vi "test Custom Regex.vi"(8 "error in":errorcluster) -> (0 "error out":errorcluster)   [LabVIEW 2020, in "serenial.io-ase.test.lvlib"]
uses:
  serenial.io-ase.test.lvlib
  Custom Regex/Custom Regex.lvclass
  C:/serenial/libraries/asynchronous-system-exec/LabVIEW/serenial.io-ase/configuration/configuration.lvclass
  serenial.io-ase/ase/ase.lvclass/ase.ctl
  serenial.io-ase/ase/Start Call (Exe-Args).vi
  serenial.io-ase/ase/Start Call (Internal).vi
  serenial.io-ase/ase/Write Data to Std In.vi
  serenial.io-ase/ase/Merge Call Library Errors.vi
  serenial.io-ase/ase/NI-Linux-RT-64 Library Path.vi
  serenial.io-ase/ase/Error Empty Executable Name.vi
  serenial.io-ase/ase/Check Shared Library Version.vi
  serenial.io-ase/ase/Trim Whitespace.vi
  serenial.io-ase/ase/Error Invalid ASE Handle.vi
  serenial.io-ase/ase/Error Internal Library Implementation Error.vi
  <vilib>/Utility/error.llb/Error Cluster From Error Code.vi
  <vilib>/addons/_JKI Toolkits/Caraya/classes/Assert/Assert Equal Value and Type_Variant.vi
  serenial.io-ase/ase/ase.lvclass
  <vilib>/ErrorRing/Error Ring.xnode
  serenial.io-ase/configuration/configuration.lvclass
  <vilib>/addons/_JKI Toolkits/Caraya/classes/Test/Test.lvclass
  <vilib>/addons/_JKI Toolkits/Caraya/classes/Assert/Assert.lvclass
  C:/serenial/libraries/asynchronous-system-exec/LabVIEW/serenial.io-ase.test/Custom Regex/Custom Regex.lvclass
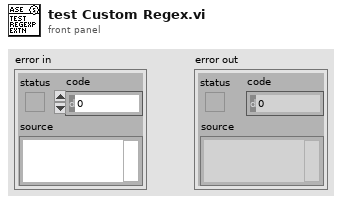
[diagram p1: front panel]
types:
  T1 = typedef "serenial.io-ase.lvlib/ase.lvclass/Event References.ctl" = cluster{"Standard Output":refnum<user-event>, "Standard Error":refnum<user-event>, "Did Exit":refnum<user-event>}
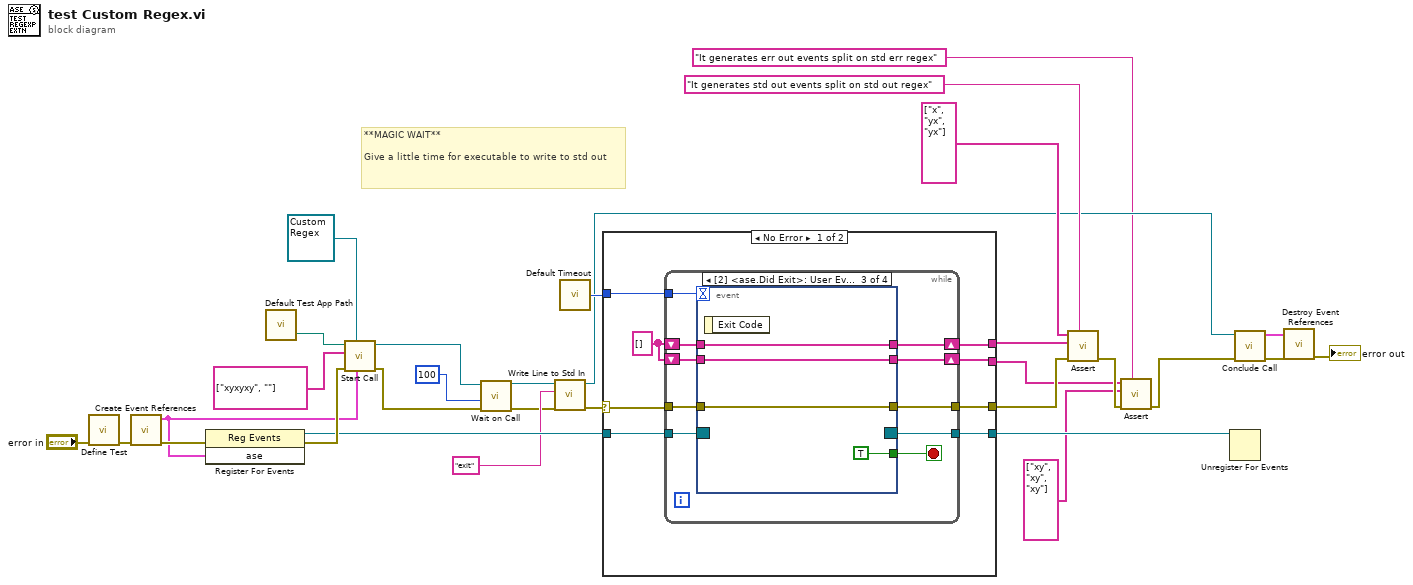
[diagram p0: block diagram]
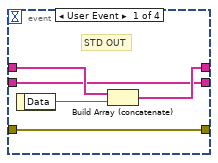
[diagram p2: hidden frame]
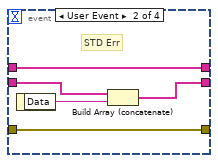
[diagram p3: hidden frame]
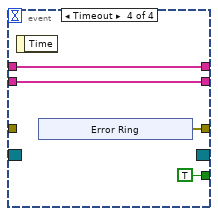
[diagram p4: hidden frame]
diagram:
  # "**MAGIC WAIT**\n\nGive a little time for executable to write to std out"
  n1 = call <vilib>:"Define Test.vi"("error in (no error)"="error in") -> ("error out"=w29:errorcluster)  [unwired: 10 in]
  n2 = call "Create Event References.vi"("error in"=w29) -> ("error out"=w31:errorcluster, "ase"=w19:T1)  [unwired: 9 in]
  n3 = register-events(error in=w31, w19) -> (reference out=w25:refnum<event-registration>, error out=w30:errorcluster)  [unwired: 1 in]
  n4 = call "Default Test App Path.vi"() -> ("Exe Path"=w6:path)  [unwired: 2 in, 1 out]
  n5 = call-poly "Start Call.vi"("Event References"=w19, "Configuration"=refnum<class "Custom Regex.lvclass"> refnum ("serenial.io-ase.test.lvlib:Custom Regex.lvclass"), "error in"=w30, "Arguments (Default: Empty)"=string[] ["xyxyxy", ""] ("Input"), "Executable Path"=w6) -> ("error out"=w4:errorcluster, "New ASE Handle"=w5:refnum<class "ase.lvclass">)  [unwired: 5 in]
  n6 = call "Wait on Call.vi"("error in"=w4, "Timeout (ms)"=100, "ASE Handle"=w5) -> ("error out"=w2:errorcluster, "ASE Handle Duplicate"=w3:refnum<class "ase.lvclass">)  [unwired: 6 in, 1 out]
  n7 = call "Write Line to Std In .vi"("error in"=w2, "Input"="exit", "ASE Handle"=w3) -> ("error out"=w27:errorcluster, "ASE Handle Duplicate"=w16:refnum<class "ase.lvclass">)  [unwired: 6 in, 1 out]
  n8 = call "Default Timeout.vi"() -> ("Default Timeout"=w20:i32)
  n9 = case shown="No Error" w27 {
    selector: w27 -> [w39 w74]
    tunnel: w25 -> [w37 w73]
    tunnel: [w36 w73] -> w24
    tunnel: [w35 _] -> w15
    tunnel: [w38 w74] -> w26
    tunnel: w20 -> [w34 _]
    tunnel: [w32 _] -> w10
    frame No Error {
      w33 = string[] []
      n10 = while {
        tunnel: w39 -> [w49]
        tunnel: w37 -> [w47]
        tunnel: [w46] -> w36
        shift-right: [w44] -> w35
        shift-left: w33 -> [w45]
        tunnel: [w48] -> w38
        tunnel: w34 -> [w43]
        shift-right: [w42] -> w32
        shift-left: w33 -> [w41]
        stop <- w40 stop-if-true
        n11 = event shown="[2] <ase.Did Exit>: User Event" {
          selector: w47 -> [_ _ _ _]
          dyn-events: [_ _ _ _] -> w46
          timeout: w43 -> [_ _ _ _]
          tunnel: w49 -> [w54 w59 w63 _]
          tunnel: [w54 w59 w63 w66] -> w48
          tunnel: w45 -> [w52 w57 w62 w67]
          tunnel: [w51 w57 w62 w67] -> w44
          tunnel: [w50 w56 w61 w65] -> w42
          tunnel: w41 -> [w50 w55 w61 w65]
          tunnel: [_ _ TRUE TRUE] -> w40
          event User Event {
            # "STD OUT"
            n12 = event-data() -> ("Data"=w53:string)  [unwired: 1 in]
            n13 = Build Array (concatenate)(w52, w53) -> (w51:string[])
          }
          event User Event {
            # "STD Err"
            n14 = event-data() -> ("Data"=w58:string)  [unwired: 1 in]
            n15 = Build Array (concatenate)(w55, w58) -> (w56:string[])
          }
          event User Event {
            n16 = event-data() -> ()  [unwired: 1 in, 1 out]
          }
          event Timeout {
            n17 = event-data() -> ()  [unwired: 1 in, 1 out]
            n18 = xnode ("Error Ring")() -> ("error out"=w66:errorcluster)
          }
        }
      }
    }
    frame Error {
    }
  }
  n19 = call-poly <vilib>:"Assert.vi"("Label"="It generates std out events split on std out regex", "error in (no error)"=w26, "Y"=w15, "X"=string[] ["x", "yx", "yx"] ("Array")) -> ("error out"=w12:errorcluster)  [unwired: 7 in]
  n20 = call-poly <vilib>:"Assert.vi"("Label"="It generates err out events split on std err regex", "error in (no error)"=w12, "Y"=string[] ["xy", "xy", "xy"] ("Array"), "X"=w10) -> ("error out"=w11:errorcluster)  [unwired: 7 in]
  n21 = Unregister For Events(event registration refnum=w24) -> ()  [unwired: 1 in, 1 out]
  n22 = call "Conclude Call.vi"("error in"=w11, "ASE Handle"=w16) -> ("error out"=w18:errorcluster, "Event References"=w14:T1)  [unwired: 7 in, 1 out]
  n23 = call "Destroy Event References.vi"("error in"=w18, "Event References"=w14) -> ("error out"=→"error out":errorcluster)  [unwired: 9 in]
